vi "Ref_FIFO Flush.vi"(8 "Error In":errorcluster, 11 "FPGA VI Ref":T1) -> (0 "Error Out":errorcluster, 3 "FPGA VI Reference Out":T1)   [LabVIEW 2017]
uses:
  RIG-SPECIFIC FILES/FPGA Refs/FPGA Ref.ctl
  <vilib>/Utility/error.llb/Error Cluster From Error Code.vi
  <vilib>/rvi/errors/niLvFpgaAdjustHostInterfaceError.vi
  <vilib>/rvi/interface/nirviMethod/nirviMethod.xnode
  <vilib>/rvi/errors/niLvFpgaMergeErrorWithErrorCode.vi
  <vilib>/FPGAPlugInAG/Dynamic/niLvFpga_ReadFifo_Dynamic.vi
panel:
  out "Data":u32[](array[numeric])
  in  "Manual force stop":bool
  out "Elements Remaining":u32
  out "Loop":i32
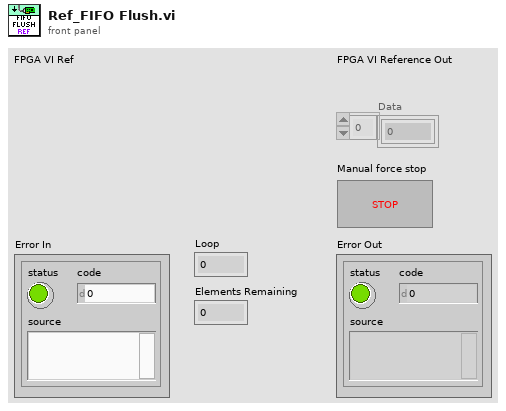
[diagram p1: front panel]
types:
  T1 = typedef "FPGA Ref.ctl" = refnum<k20>
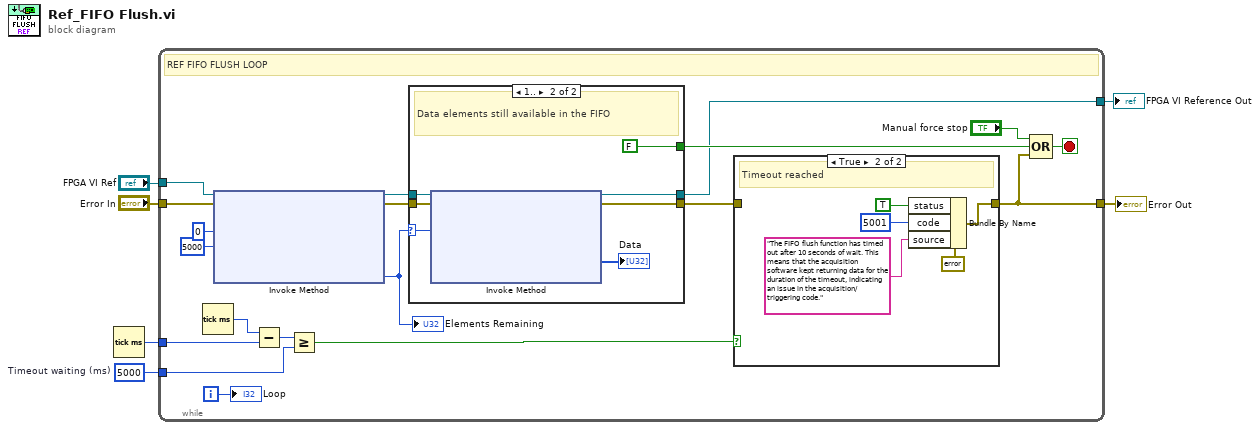
[diagram p0: block diagram]
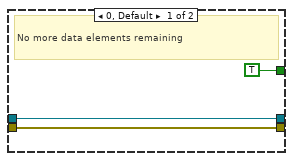
[diagram p3: hidden frame]
diagram:
  w4 = u32 5000  # Timeout waiting (ms)
  n1 = Tick Count (ms)() -> (millisecond timer value=w3:u32)
  n2 = while {
    tunnel: "FPGA VI Ref" -> [w8]
    tunnel: "Error In" -> [w25]
    tunnel: [w10] -> w5
    tunnel: w3 -> [w17]
    tunnel: w4 -> [w13]
    tunnel: [w7] -> w1
    i -> [w24]
    stop <- w23 stop-if-true
    # "REF FIFO FLUSH LOOP"
    n3 = Tick Count (ms)() -> (millisecond timer value=w18:u32)
    n4 = xnode "Invoke Method"("FPGA VI Reference In"=w8, "error in"=w25, "Number of Elements"=u32 0, "Timeout (ms)"=5000) -> ("FPGA VI Reference Out"=w21:T1, "error out"=w22:errorcluster, "Elements Remaining"=w16:u32)  [unwired: 1 out]
    "Elements Remaining" <- w16
    n5 = Subtract(x=w18, y=w17) -> (x-y=w14:u32)
    n6 = Greater Or Equal?(x=w14, y=w13) -> (x >= y?=w12:bool)
    n7 = case shown="1.." w16 {
      selector: w16 -> [_ w38]
      tunnel: w22 -> [w33 w41]
      tunnel: w21 -> [w32 w40]
      tunnel: [w33 w39] -> w11
      tunnel: [TRUE FALSE] -> w15
      tunnel: [w32 w35] -> w7
      frame 0, Default {
        # "No more data elements remaining"
      }
      frame 1.. {
        # "Data elements still available in the FIFO"
        n8 = xnode "Invoke Method"("FPGA VI Reference In"=w40, "error in"=w41, "Number of Elements"=w38) -> ("FPGA VI Reference Out"=w35:T1, "error out"=w39:errorcluster, "Data"=→"Data":u16[])  [unwired: 1 in, 1 out]
      }
    }
    n9 = case shown="True" w12 {
      tunnel: w11 -> [w26 _]
      tunnel: [w26 w27] -> w10
      frame False {
      }
      frame True {
        # "Timeout reached"
        n10 = Bundle By Name(cluster=errorcluster {"status"=TRUE, "code"=5001, "source"=""} ("error out"), "status"=TRUE, "code"=5001, "source"="The FIFO flush function has timed out after 10 seconds of wait. This means that the acquisition software kept returning data for the duration of the timeout, indicating an issue in the acquisition/triggering code." ("Error Source")) -> (w27:errorcluster)
      }
    }
    n11 = Compound Arithmetic op=OR("Manual force stop", w15, w10) -> (w23:bool)
    "Loop" <- w24
  }
  "Error Out" <- w5
  "FPGA VI Reference Out" <- w1
